vi "criteria_count.vi"(5 "change_in_event":refnum<user-event>, 7 "waitgroup":T1, 8 "error in (no error)":errorcluster, 10 "recipe_data":variant, 11 "criteria":variant) -> (0 "error out":errorcluster)   [LabVIEW 2015, in "example_01.lvlib"]
uses:
  example_01.lvlib
  <userlib>/antonio-alexander/lv-waitgroup/public/_controls/api_waitgroup.ctl
  lv-recipe-machine/public/_controls/change.ctl
  _controls/recipes.ctl
  _controls/steps_actions_data.ctl
  _controls/steps_actions.ctl
  lv-recipe-machine/lv-recipe-machine.lvlib
  <userlib>/antonio-alexander/lv-waitgroup/lv-waitgroup.lvlib
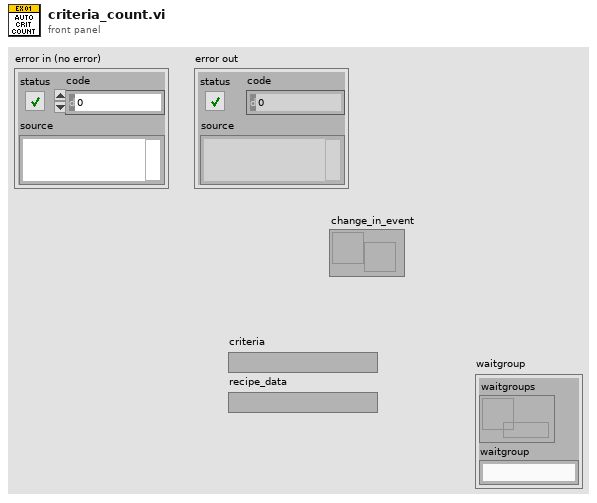
[diagram p1: front panel]
types:
  T1 = typedef "lv-waitgroup.lvlib/api_waitgroup.ctl" = cluster{"waitgroups":refnum<data-value>, "waitgroup":string}
  T2 = typedef "example_01.lvlib/recipes.ctl" = enum16{"<recipes>", "wait_random", "random_wait", "count", "comparison", "<null>"}
  T3 = typedef "example_01.lvlib/steps_actions.ctl" = enum16{"<steps_actions>", "manual_random", "manual_comparison", "manual_wait", "auto_random", "auto_wait", "criteria_initialize", "criteria_count", "criteria_comparison", "transition_simple", "transition_count", "transition_comparison", "<null>"}
  T4 = typedef "example_01.lvlib/steps_actions_data.ctl" = cluster{"step_action":T3, "data":variant}
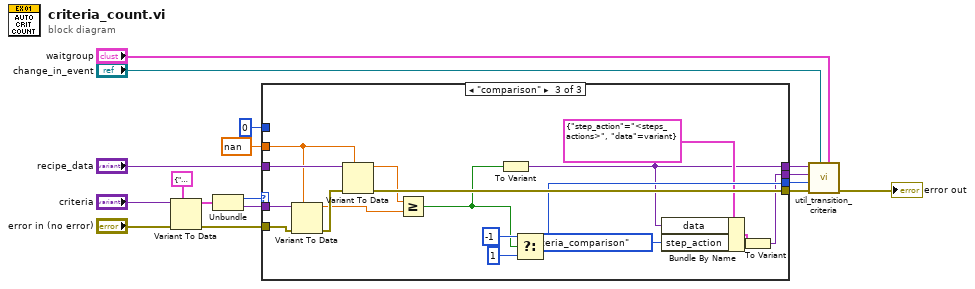
[diagram p0: block diagram]
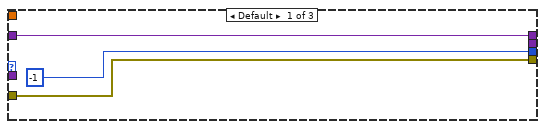
[diagram p2: hidden frame]
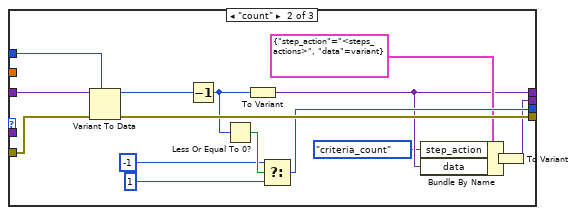
[diagram p3: hidden frame]
diagram:
  n1 = Variant To Data(error in="error in (no error)", type=cluster{"recipe":T2, variant} {"recipe"=enum."<recipes>", variant}, Variant="criteria") -> (data=w13:cluster{"recipe":T2, variant}, error out=w9:errorcluster)
  n2 = Unbundle(w13) -> ("recipe"=w11:T2, w3:variant)
  n3 = case shown="\"comparison\"" w11 {
    tunnel: w9 -> [w19 w31 w46]
    tunnel: "recipe_data" -> [w20 w35 w52]
    tunnel: [w20 w24 w37] -> w4
    tunnel: [w19 w34 w51] -> w5
    tunnel: 0 -> [_ w33 _]
    tunnel: nan -> [_ _ w45]
    tunnel: w3 -> [_ _ w47]
    tunnel: [-1 w29 w50] -> w2
    tunnel: [_ w21 w38] -> w1
    frame Default {
    }
    frame "count" {
      n4 = Variant To Data(error in=w31, type=w33, Variant=w35) -> (data=w32:i32, error out=w34:errorcluster)
      n5 = Decrement(x=w32) -> (x-1=w30:i32)
      n6 = Less Or Equal To 0?(x=w30) -> (x <= 0?=w28:bool)
      n7 = To Variant(anything=w30) -> (Variant=w24:variant)
      n8 = Select(t=-1, s=w28, f=1) -> (s? t:f=w29:i32)
      n9 = Bundle By Name(cluster=T4 {"step_action"=enum."<steps_actions>", "data"=variant} ("step_data"), "step_action"=steps_actions."criteria_count", "data"=w24) -> (w22:T4)
      n10 = To Variant(anything=w22) -> (Variant=w21:variant)
    }
    frame "comparison" {
      n11 = Variant To Data(error in=w46, type=w45, Variant=w47) -> (data=w42:dbl, error out=w44:errorcluster)
      n12 = Variant To Data(error in=w44, type=w45, Variant=w52) -> (data=w43:dbl, error out=w51:errorcluster)
      n13 = Greater Or Equal?(x=w43, y=w42) -> (x >= y?=w41:bool)
      n14 = To Variant(anything=w41) -> (Variant=w37:variant)
      n15 = Select(t=-1, s=w41, f=1) -> (s? t:f=w50:i32)
      n16 = Bundle By Name(cluster=T4 {"step_action"=enum."<steps_actions>", "data"=variant} ("step_data"), "data"=w37, "step_action"=steps_actions."criteria_comparison") -> (w39:T4)
      n17 = To Variant(anything=w39) -> (Variant=w38:variant)
    }
  }
  n18 = call "util_transition_criteria.vi"("api_waitgroup"="waitgroup", "change_in_event"="change_in_event", "error in (no error)"=w5, "next_index"=w2, "data"=w1, "recipe_data"=w4) -> ("error out"=→"error out":errorcluster)  [unwired: 5 in]
